vi "Swerve Begin.vi"(8 "BR Drive Invert":bool, 9 "BL Drive Invert":bool, 10 "FR Drive Invert":bool, 11 "FL Drive Invert":bool) -> ()   [LabVIEW 2017]
uses:
  <vilib>/Rock Robotics/WPI/ThirdParty/Phoenix-LabVIEW/Motor Controller/Controls/CTRE_Phoenix_MotorControl_NeutralMode.ctl
  <vilib>/Rock Robotics/WPI/ThirdParty/Phoenix-LabVIEW/Motor Controller/Controls/CTRE_Phoenix_MotorControl_FeedbackDevice.ctl
  <vilib>/Rock Robotics/SystemInterfaces/DIO/FPGA_DIOPWMChannel.ctl
  <vilib>/Rock Robotics/WPI/SafetyOutput/WPI_SafetyOutputConfigMenu.ctl
  <vilib>/Rock Robotics/WPI/MotorControl/WPI_MotorControlOpen VictorSP.vi
  Robot Global Data.vi
  <vilib>/Utility/file.llb/Read Delimited Spreadsheet (DBL).vi
  <vilib>/Rock Robotics/Network Tables/NT Write Numeric Array.vi
panel:
  in  "Feedback Device":T1=8 items=["None"=-1, "QuadEncoder"=0, "Analog"=2, "Tachometer"=4, "Pulse Width Encoded Position"=8, "Sensor Sum (S0 + S1)"=9, "Sensor Difference (D0 - D1)"=10, "Remote Source 0"=11, "Remote Source 1"=12, "Software Emulated"=15]
  in  "allowableClosedLoopError":i32=50
  in  "Ramp Rate":dbl=0.15
  in  "Motor B/C Mode":T2=enum."Override to Coast"
  # "Value in Seconds"
  # "Raw Units Only\nSensor Resoution is 1 Rotation = 4096 units"
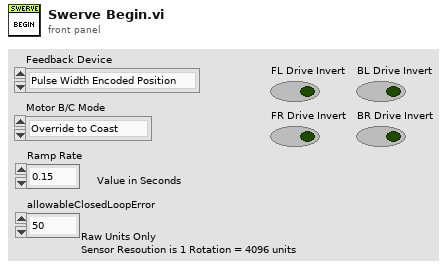
[diagram p1: front panel]
types:
  T1 = typedef "CTRE_Phoenix_MotorControl_FeedbackDevice.ctl" = i8
  T2 = typedef "CTRE_Phoenix_MotorControl_NeutralMode.ctl" = enum8{"EEPROMSetting", "Override to Coast", "Override to Brake"}
  T3 = typedef "WPI_SafetyOutputConfigMenu.ctl" = enum16{"Enable", "Disable"}
  T4 = typedef "FPGA_DIOPWMChannel.ctl" = enum8{"PWM 0", "PWM 1", "PWM 2", "PWM 3", "PWM 4", "PWM 5", "PWM 6", "PWM 7", "PWM 8", "PWM 9", "PWM MXP 0", "PWM MXP 1", "PWM MXP 2", "PWM MXP 3", "PWM MXP 4", "PWM MXP 5", "PWM MXP 6", "PWM MXP 7", "PWM MXP 8", "PWM MXP 9", "Invalid"}
  T5 = typedef "WPI_MotorControlDeviceRef.ctl" = cluster{"DeviceStatus":errorcluster, "Type":T6, "PWM":cluster{"PWM Channel":T4, "DeadBand":T7}, "CAN":cluster{"Device Number":u8, "SetOutput VI Ref":variant, "GetOutput VI Ref":variant, "Enable VI Ref":variant, "Disable VI Ref":variant, "Data":variant}, "Invert":bool, "DIO PWM":cluster{"PWM \"Enable\" Channel":T4, "DIOChannel":T8, "PWM Rate":dbl}}
  T6 = typedef "WPI_MotorControlType.ctl" = enum16{"PWM", "CAN", "DIO PWM"}
  T7 = typedef "WPI_PWMDeadband.ctl" = cluster{"Name":string, "maxPositivePwm":i32, "minPositivePwm":i32, "centerPwm":i32, "maxNegativePwm":i32, "minNegativePwm":i32, "angularRange":u16}
  T8 = typedef "FPGA_DIOChannel.ctl" = enum8{"DIO 0", "DIO 1", "DIO 2", "DIO 3", "DIO 4", "DIO 5", "DIO 6", "DIO 7", "DIO 8", "DIO 9", "DIO MXP 0", "DIO MXP 1", "DIO MXP 2", "DIO MXP 3", "DIO MXP 4", "DIO MXP 5", "DIO MXP 6", "DIO MXP 7", "DIO MXP 8", "DIO MXP 9", "DIO MXP 10", "DIO MXP 11", "DIO MXP 12", "DIO MXP 13", "DIO MXP 14", "DIO MXP 15", "SPI Port CS1", "SPI Port CS2", "SPI Port CS3", "SPI Port MISO", "SPI Port MOSI", "Invalid"}
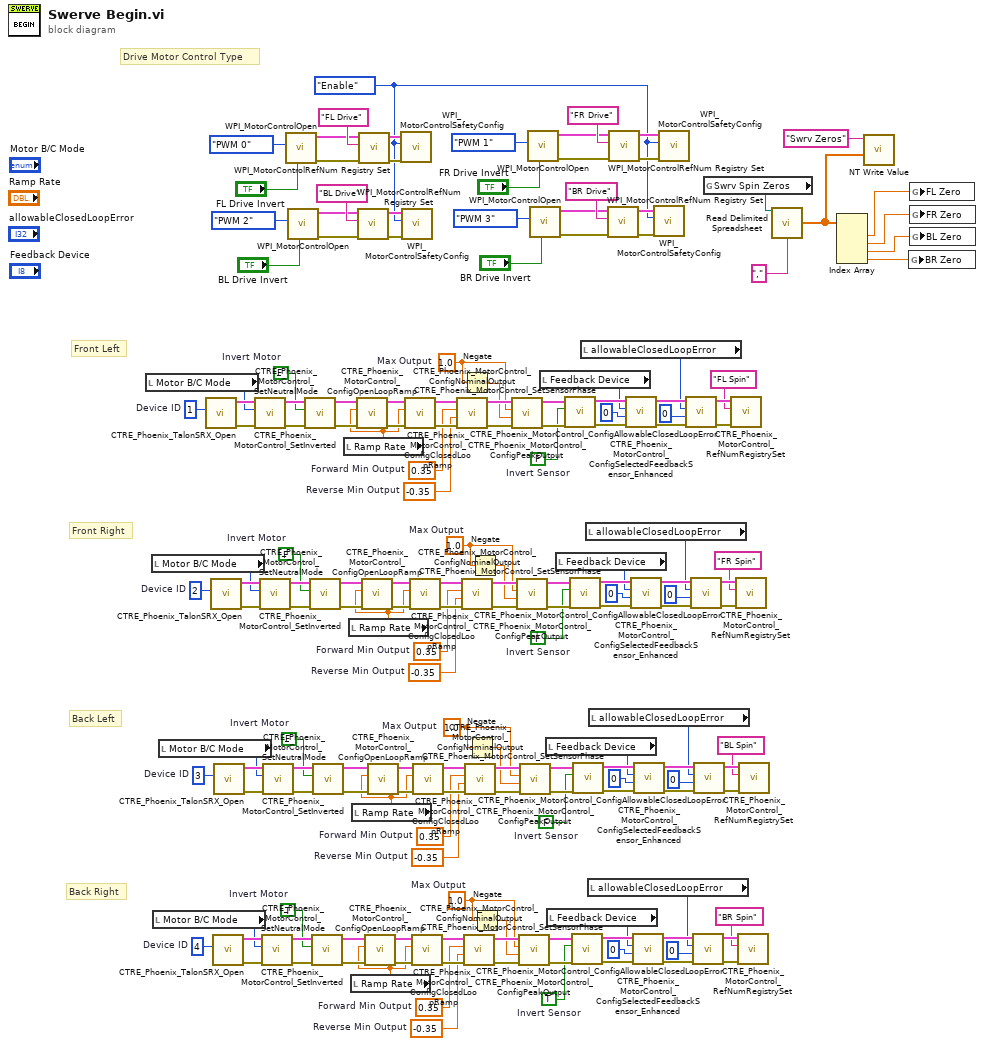
[diagram p0: block diagram]
diagram:
  w5 = WPI_SafetyOutputConfigMenu."Enable" ("mode")
  w17 = 1.0  # Max Output
  w19 = 1.0  # Max Output
  w21 = 1.0  # Max Output
  w55 = -0.35  # Reverse Min Output
  w54 = 0.35  # Forward Min Output
  w61 = TRUE  # Invert Motor
  w70 = TRUE  # Invert Sensor
  w79 = u8 4  # Device ID
  w81 = -0.35  # Reverse Min Output
  w80 = 0.35  # Forward Min Output
  w87 = FALSE  # Invert Motor
  w96 = FALSE  # Invert Sensor
  w105 = u8 3  # Device ID
  w107 = -0.35  # Reverse Min Output
  w106 = 0.35  # Forward Min Output
  w113 = FALSE  # Invert Motor
  w122 = FALSE  # Invert Sensor
  w131 = u8 2  # Device ID
  w133 = -0.35  # Reverse Min Output
  w132 = 0.35  # Forward Min Output
  w22 = 1.0  # Max Output
  w139 = FALSE  # Invert Motor
  w148 = FALSE  # Invert Sensor
  w157 = u8 1  # Device ID
  # "Front Left"
  # "Front Right"
  # "Back Left"
  # "Back Right"
  # "Drive Motor Control Type"
  n1 = local read "Motor B/C Mode"() -> (w135:T2)
  n2 = local read "Motor B/C Mode"() -> (w109:T2)
  n3 = local read "Motor B/C Mode"() -> (w57:T2)
  n4 = local read "Motor B/C Mode"() -> (w83:T2)
  n5 = call <vilib>:"CTRE_Phoenix_TalonSRX_Open.vi"("Device Number"=w157) -> ("error out"=w156:errorcluster, "CAN Talon SRX Ref"=w155:T5)  [unwired: 9 in]
  n6 = call <vilib>:"CTRE_Phoenix_TalonSRX_Open.vi"("Device Number"=w131) -> ("error out"=w130:errorcluster, "CAN Talon SRX Ref"=w129:T5)  [unwired: 9 in]
  n7 = call <vilib>:"CTRE_Phoenix_TalonSRX_Open.vi"("Device Number"=w79) -> ("error out"=w78:errorcluster, "CAN Talon SRX Ref"=w77:T5)  [unwired: 9 in]
  n8 = call <vilib>:"CTRE_Phoenix_TalonSRX_Open.vi"("Device Number"=w105) -> ("error out"=w104:errorcluster, "CAN Talon SRX Ref"=w103:T5)  [unwired: 9 in]
  n9 = call <vilib>:"CTRE_Phoenix_MotorControl_SetNeutralMode.vi"("error in (no error)"=w156, "Motor Control Neutral Mode"=w135, "PhoenixMotorControlDevRef"=w155) -> ("error out"=w140:errorcluster, "PhoenixMotorControlDevRef"=w141:T5)  [unwired: 7 in]
  n10 = call <vilib>:"CTRE_Phoenix_MotorControl_SetNeutralMode.vi"("error in (no error)"=w130, "Motor Control Neutral Mode"=w109, "PhoenixMotorControlDevRef"=w129) -> ("error out"=w114:errorcluster, "PhoenixMotorControlDevRef"=w115:T5)  [unwired: 7 in]
  n11 = call <vilib>:"CTRE_Phoenix_MotorControl_SetNeutralMode.vi"("error in (no error)"=w78, "Motor Control Neutral Mode"=w57, "PhoenixMotorControlDevRef"=w77) -> ("error out"=w62:errorcluster, "PhoenixMotorControlDevRef"=w63:T5)  [unwired: 7 in]
  n12 = call <vilib>:"CTRE_Phoenix_MotorControl_SetNeutralMode.vi"("error in (no error)"=w104, "Motor Control Neutral Mode"=w83, "PhoenixMotorControlDevRef"=w103) -> ("error out"=w88:errorcluster, "PhoenixMotorControlDevRef"=w89:T5)  [unwired: 7 in]
  n13 = call-poly <vilib>:"WPI_MotorControlOpen.vi"("Invert"="FL Drive Invert", "PWM Channel"=FPGA_DIOPWMChannel."PWM 0") -> ("error out"=w168:errorcluster, "MotorControlDeviceRef"=w169:T5)  [unwired: 8 in]
  n14 = call-poly <vilib>:"WPI_MotorControlOpen.vi"("Invert"="BL Drive Invert", "PWM Channel"=FPGA_DIOPWMChannel."PWM 2") -> ("error out"=w162:errorcluster, "MotorControlDeviceRef"=w163:T5)  [unwired: 8 in]
  n15 = call <vilib>:"CTRE_Phoenix_MotorControl_SetInverted.vi"("error in (no error)"=w140, "Invert?"=w139, "PhoenixMotorControlDevRef"=w141) -> ("error out"=w53:errorcluster, "PhoenixMotorControlDevRef"=w52:T5)  [unwired: 7 in]
  n16 = call <vilib>:"CTRE_Phoenix_MotorControl_SetInverted.vi"("error in (no error)"=w114, "Invert?"=w113, "PhoenixMotorControlDevRef"=w115) -> ("error out"=w46:errorcluster, "PhoenixMotorControlDevRef"=w47:T5)  [unwired: 7 in]
  n17 = call <vilib>:"CTRE_Phoenix_MotorControl_SetInverted.vi"("error in (no error)"=w62, "Invert?"=w61, "PhoenixMotorControlDevRef"=w63) -> ("error out"=w38:errorcluster, "PhoenixMotorControlDevRef"=w39:T5)  [unwired: 7 in]
  n18 = call <vilib>:"CTRE_Phoenix_MotorControl_SetInverted.vi"("error in (no error)"=w88, "Invert?"=w87, "PhoenixMotorControlDevRef"=w89) -> ("error out"=w42:errorcluster, "PhoenixMotorControlDevRef"=w43:T5)  [unwired: 7 in]
  n19 = local read "Ramp Rate"() -> (w34:dbl)
  n20 = local read "Ramp Rate"() -> (w35:dbl)
  n21 = local read "Ramp Rate"() -> (w37:dbl)
  n22 = local read "Ramp Rate"() -> (w36:dbl)
  n23 = call <vilib>:"CTRE_Phoenix_MotorControl_ConfigOpenLoopRamp.vi"("error in (no error)"=w53, "secondsFromNeutralToFull"=w34, "PhoenixMotorControlDevRef"=w52) -> ("error out"=w50:errorcluster, "PhoenixMotorControlDevRef"=w51:T5)  [unwired: 7 in]
  n24 = call <vilib>:"WPI_MotorControlRefNum Registry Set.vi"("error in (no error)"=w162, "refnum name"="BL Drive", "MotorControlDevRef"=w163) -> ("error out"=w11:errorcluster, "MotorControlDevRef"=w10:T5)  [unwired: 7 in]
  n25 = call <vilib>:"WPI_MotorControlRefNum Registry Set.vi"("error in (no error)"=w168, "refnum name"="FL Drive", "MotorControlDevRef"=w169) -> ("error out"=w13:errorcluster, "MotorControlDevRef"=w12:T5)  [unwired: 7 in]
  n26 = call <vilib>:"CTRE_Phoenix_MotorControl_ConfigOpenLoopRamp.vi"("error in (no error)"=w46, "secondsFromNeutralToFull"=w35, "PhoenixMotorControlDevRef"=w47) -> ("error out"=w49:errorcluster, "PhoenixMotorControlDevRef"=w48:T5)  [unwired: 7 in]
  n27 = call <vilib>:"CTRE_Phoenix_MotorControl_ConfigOpenLoopRamp.vi"("error in (no error)"=w38, "secondsFromNeutralToFull"=w37, "PhoenixMotorControlDevRef"=w39) -> ("error out"=w41:errorcluster, "PhoenixMotorControlDevRef"=w40:T5)  [unwired: 7 in]
  n28 = call <vilib>:"CTRE_Phoenix_MotorControl_ConfigOpenLoopRamp.vi"("error in (no error)"=w42, "secondsFromNeutralToFull"=w36, "PhoenixMotorControlDevRef"=w43) -> ("error out"=w45:errorcluster, "PhoenixMotorControlDevRef"=w44:T5)  [unwired: 7 in]
  n29 = call <vilib>:"WPI_MotorControlSafetyConfig.vi"("error in (no error)"=w13, "mode"=w5, "MotorControlDevRef"=w12) -> ()  [unwired: 7 in, 2 out]
  n30 = call <vilib>:"WPI_MotorControlSafetyConfig.vi"("error in (no error)"=w11, "mode"=w5, "MotorControlDevRef"=w10) -> ()  [unwired: 7 in, 2 out]
  n31 = call <vilib>:"CTRE_Phoenix_MotorControl_ConfigClosedLoopRamp.vi"("error in (no error)"=w50, "secondsFromNeutralToFull"=w34, "PhoenixMotorControlDevRef"=w51) -> ("error out"=w154:errorcluster, "PhoenixMotorControlDevRef"=w153:T5)  [unwired: 7 in]
  n32 = call <vilib>:"CTRE_Phoenix_MotorControl_ConfigClosedLoopRamp.vi"("error in (no error)"=w49, "secondsFromNeutralToFull"=w35, "PhoenixMotorControlDevRef"=w48) -> ("error out"=w128:errorcluster, "PhoenixMotorControlDevRef"=w127:T5)  [unwired: 7 in]
  n33 = call <vilib>:"CTRE_Phoenix_MotorControl_ConfigClosedLoopRamp.vi"("error in (no error)"=w41, "secondsFromNeutralToFull"=w37, "PhoenixMotorControlDevRef"=w40) -> ("error out"=w76:errorcluster, "PhoenixMotorControlDevRef"=w75:T5)  [unwired: 7 in]
  n34 = call <vilib>:"CTRE_Phoenix_MotorControl_ConfigClosedLoopRamp.vi"("error in (no error)"=w45, "secondsFromNeutralToFull"=w36, "PhoenixMotorControlDevRef"=w44) -> ("error out"=w102:errorcluster, "PhoenixMotorControlDevRef"=w101:T5)  [unwired: 7 in]
  n35 = call <vilib>:"CTRE_Phoenix_MotorControl_ConfigNominalOutput.vi"("error in (no error)"=w154, "Reverse Nominal Percent Output"=w133, "Forward Nominal Percent Output"=w132, "PhoenixMotorControlDevRef"=w153) -> ("error out"=w152:errorcluster, "PhoenixMotorControlDevRef"=w151:T5)  [unwired: 6 in]
  n36 = Negate(x=w22) -> (-x=w23:dbl)
  n37 = call <vilib>:"CTRE_Phoenix_MotorControl_ConfigNominalOutput.vi"("error in (no error)"=w128, "Reverse Nominal Percent Output"=w107, "Forward Nominal Percent Output"=w106, "PhoenixMotorControlDevRef"=w127) -> ("error out"=w126:errorcluster, "PhoenixMotorControlDevRef"=w125:T5)  [unwired: 6 in]
  n38 = call <vilib>:"CTRE_Phoenix_MotorControl_ConfigNominalOutput.vi"("error in (no error)"=w76, "Reverse Nominal Percent Output"=w55, "Forward Nominal Percent Output"=w54, "PhoenixMotorControlDevRef"=w75) -> ("error out"=w74:errorcluster, "PhoenixMotorControlDevRef"=w73:T5)  [unwired: 6 in]
  n39 = call <vilib>:"CTRE_Phoenix_MotorControl_ConfigNominalOutput.vi"("error in (no error)"=w102, "Reverse Nominal Percent Output"=w81, "Forward Nominal Percent Output"=w80, "PhoenixMotorControlDevRef"=w101) -> ("error out"=w100:errorcluster, "PhoenixMotorControlDevRef"=w99:T5)  [unwired: 6 in]
  n40 = Negate(x=w19) -> (-x=w18:dbl)
  n41 = Negate(x=w21) -> (-x=w20:dbl)
  n42 = Negate(x=w17) -> (-x=w16:dbl)
  n43 = call <vilib>:"CTRE_Phoenix_MotorControl_ConfigPeakOutput.vi"("error in (no error)"=w152, "Reverse Peak Percent Output"=w23, "Forward Peak Percent Output"=w22, "PhoenixMotorControlDevRef"=w151) -> ("error out"=w150:errorcluster, "PhoenixMotorControlDevRef"=w149:T5)  [unwired: 6 in]
  n44 = call <vilib>:"CTRE_Phoenix_MotorControl_ConfigPeakOutput.vi"("error in (no error)"=w126, "Reverse Peak Percent Output"=w20, "Forward Peak Percent Output"=w21, "PhoenixMotorControlDevRef"=w125) -> ("error out"=w124:errorcluster, "PhoenixMotorControlDevRef"=w123:T5)  [unwired: 6 in]
  n45 = call <vilib>:"CTRE_Phoenix_MotorControl_ConfigPeakOutput.vi"("error in (no error)"=w74, "Reverse Peak Percent Output"=w16, "Forward Peak Percent Output"=w17, "PhoenixMotorControlDevRef"=w73) -> ("error out"=w72:errorcluster, "PhoenixMotorControlDevRef"=w71:T5)  [unwired: 6 in]
  n46 = call <vilib>:"CTRE_Phoenix_MotorControl_ConfigPeakOutput.vi"("error in (no error)"=w100, "Reverse Peak Percent Output"=w18, "Forward Peak Percent Output"=w19, "PhoenixMotorControlDevRef"=w99) -> ("error out"=w98:errorcluster, "PhoenixMotorControlDevRef"=w97:T5)  [unwired: 6 in]
  n47 = call-poly <vilib>:"WPI_MotorControlOpen.vi"("Invert"="FR Drive Invert", "PWM Channel"=FPGA_DIOPWMChannel."PWM 1") -> ("error out"=w158:errorcluster, "MotorControlDeviceRef"=w159:T5)  [unwired: 8 in]
  n48 = call-poly <vilib>:"WPI_MotorControlOpen.vi"("Invert"="BR Drive Invert", "PWM Channel"=FPGA_DIOPWMChannel."PWM 3") -> ("error out"=w160:errorcluster, "MotorControlDeviceRef"=w161:T5)  [unwired: 8 in]
  n49 = local read "Feedback Device"() -> (w33:T1)
  n50 = local read "Feedback Device"() -> (w31:T1)
  n51 = local read "Feedback Device"() -> (w30:T1)
  n52 = local read "Feedback Device"() -> (w32:T1)
  n53 = call <vilib>:"CTRE_Phoenix_MotorControl_SetSensorPhase.vi"("error in (no error)"=w150, "PhaseSensor"=w148, "PhoenixMotorControlDevRef"=w149) -> ("error out"=w147:errorcluster, "PhoenixMotorControlDevRef"=w146:T5)  [unwired: 7 in]
  n54 = call <vilib>:"CTRE_Phoenix_MotorControl_SetSensorPhase.vi"("error in (no error)"=w124, "PhaseSensor"=w122, "PhoenixMotorControlDevRef"=w123) -> ("error out"=w121:errorcluster, "PhoenixMotorControlDevRef"=w120:T5)  [unwired: 7 in]
  n55 = call <vilib>:"CTRE_Phoenix_MotorControl_SetSensorPhase.vi"("error in (no error)"=w72, "PhaseSensor"=w70, "PhoenixMotorControlDevRef"=w71) -> ("error out"=w69:errorcluster, "PhoenixMotorControlDevRef"=w68:T5)  [unwired: 7 in]
  n56 = call <vilib>:"CTRE_Phoenix_MotorControl_SetSensorPhase.vi"("error in (no error)"=w98, "PhaseSensor"=w96, "PhoenixMotorControlDevRef"=w97) -> ("error out"=w95:errorcluster, "PhoenixMotorControlDevRef"=w94:T5)  [unwired: 7 in]
  n57 = local read "allowableClosedLoopError"() -> (w134:i32)
  n58 = local read "allowableClosedLoopError"() -> (w108:i32)
  n59 = local read "allowableClosedLoopError"() -> (w56:i32)
  n60 = local read "allowableClosedLoopError"() -> (w82:i32)
  n61 = call <vilib>:"WPI_MotorControlRefNum Registry Set.vi"("error in (no error)"=w160, "refnum name"="BR Drive", "MotorControlDevRef"=w161) -> ("error out"=w9:errorcluster, "MotorControlDevRef"=w8:T5)  [unwired: 7 in]
  n62 = call <vilib>:"WPI_MotorControlRefNum Registry Set.vi"("error in (no error)"=w158, "refnum name"="FR Drive", "MotorControlDevRef"=w159) -> ("error out"=w7:errorcluster, "MotorControlDevRef"=w6:T5)  [unwired: 7 in]
  n63 = call <vilib>:"CTRE_Phoenix_MotorControl_ConfigSelectedFeedbackSensor_Enhanced.vi"("error in (no error)"=w147, "pidLoopIdx"=0, "Feedback Device"=w33, "PhoenixMotorControlDevRef"=w146) -> ("error out"=w144:errorcluster, "PhoenixMotorControlDevRef"=w143:T5)  [unwired: 6 in]
  n64 = call <vilib>:"CTRE_Phoenix_MotorControl_ConfigSelectedFeedbackSensor_Enhanced.vi"("error in (no error)"=w121, "pidLoopIdx"=0, "Feedback Device"=w32, "PhoenixMotorControlDevRef"=w120) -> ("error out"=w118:errorcluster, "PhoenixMotorControlDevRef"=w117:T5)  [unwired: 6 in]
  n65 = call <vilib>:"CTRE_Phoenix_MotorControl_ConfigSelectedFeedbackSensor_Enhanced.vi"("error in (no error)"=w69, "pidLoopIdx"=0, "Feedback Device"=w30, "PhoenixMotorControlDevRef"=w68) -> ("error out"=w66:errorcluster, "PhoenixMotorControlDevRef"=w65:T5)  [unwired: 6 in]
  n66 = call <vilib>:"CTRE_Phoenix_MotorControl_ConfigSelectedFeedbackSensor_Enhanced.vi"("error in (no error)"=w95, "pidLoopIdx"=0, "Feedback Device"=w31, "PhoenixMotorControlDevRef"=w94) -> ("error out"=w92:errorcluster, "PhoenixMotorControlDevRef"=w91:T5)  [unwired: 6 in]
  n67 = call <vilib>:"WPI_MotorControlSafetyConfig.vi"("error in (no error)"=w9, "mode"=w5, "MotorControlDevRef"=w8) -> ()  [unwired: 7 in, 2 out]
  n68 = call <vilib>:"WPI_MotorControlSafetyConfig.vi"("error in (no error)"=w7, "mode"=w5, "MotorControlDevRef"=w6) -> ()  [unwired: 7 in, 2 out]
  n69 = call <vilib>:"CTRE_Phoenix_MotorControl_ConfigAllowableClosedLoopError.vi"("error in (no error)"=w144, "slotIdx"=u32 0, "allowableClosedLoopError"=w134, "PhoenixMotorControlDevRef"=w143) -> ("error out"=w138:errorcluster, "PhoenixMotorControlDevRef"=w137:T5)  [unwired: 6 in]
  n70 = call <vilib>:"CTRE_Phoenix_MotorControl_ConfigAllowableClosedLoopError.vi"("error in (no error)"=w118, "slotIdx"=u32 0, "allowableClosedLoopError"=w108, "PhoenixMotorControlDevRef"=w117) -> ("error out"=w112:errorcluster, "PhoenixMotorControlDevRef"=w111:T5)  [unwired: 6 in]
  n71 = call <vilib>:"CTRE_Phoenix_MotorControl_ConfigAllowableClosedLoopError.vi"("error in (no error)"=w66, "slotIdx"=u32 0, "allowableClosedLoopError"=w56, "PhoenixMotorControlDevRef"=w65) -> ("error out"=w60:errorcluster, "PhoenixMotorControlDevRef"=w59:T5)  [unwired: 6 in]
  n72 = call <vilib>:"CTRE_Phoenix_MotorControl_ConfigAllowableClosedLoopError.vi"("error in (no error)"=w92, "slotIdx"=u32 0, "allowableClosedLoopError"=w82, "PhoenixMotorControlDevRef"=w91) -> ("error out"=w86:errorcluster, "PhoenixMotorControlDevRef"=w85:T5)  [unwired: 6 in]
  n73 = global read "Robot Global Data.vi" "Swrv Spin Zeros"() -> (w24:path)
  n74 = call <vilib>:"CTRE_Phoenix_MotorControl_RefNumRegistrySet.vi"("error in (no error)"=w138, "refnum name"="FL Spin", "PhoenixMotorControlDevRef"=w137) -> ()  [unwired: 7 in, 2 out]
  n75 = call <vilib>:"CTRE_Phoenix_MotorControl_RefNumRegistrySet.vi"("error in (no error)"=w112, "refnum name"="FR Spin", "PhoenixMotorControlDevRef"=w111) -> ()  [unwired: 7 in, 2 out]
  n76 = call <vilib>:"CTRE_Phoenix_MotorControl_RefNumRegistrySet.vi"("error in (no error)"=w60, "refnum name"="BR Spin", "PhoenixMotorControlDevRef"=w59) -> ()  [unwired: 7 in, 2 out]
  n77 = call <vilib>:"CTRE_Phoenix_MotorControl_RefNumRegistrySet.vi"("error in (no error)"=w86, "refnum name"="BL Spin", "PhoenixMotorControlDevRef"=w85) -> ()  [unwired: 7 in, 2 out]
  n78 = call-poly <vilib>:"Read Delimited Spreadsheet.vi"("file path (dialog if empty)"=w24, "delimiter (\\t)"="," ("delimiter (\\t)")) -> ("first row"=w14:dbl[])  [unwired: 8 in, 5 out]
  n79 = Index Array(array=w14) -> (element #1=w25:dbl, element #2=w26:dbl, element #3=w27:dbl, element #4=w28:dbl)  [unwired: 4 in]
  n80 = call-poly <vilib>:"NT Write Value.vi"("Numeric Array"=w14, "Name"="Swrv Zeros") -> ()  [unwired: 9 in, 1 out]
  n81 = global write "Robot Global Data.vi" "BR Zero"(w28) -> ()
  n82 = global write "Robot Global Data.vi" "FL Zero"(w25) -> ()
  n83 = global write "Robot Global Data.vi" "FR Zero"(w26) -> ()
  n84 = global write "Robot Global Data.vi" "BL Zero"(w27) -> ()
